vi "5668 Close Scan with External LO.vi"(8 "error in (no error)":errorcluster, 11 "Instrument Handles in":T1={"Resource Name RFSA"="RFSA", "Resource Name RFSG LO Generation"="RFSG"}) -> (0 "error out":errorcluster)   [LabVIEW 2017]
uses:
  Instrument Handles.ctl
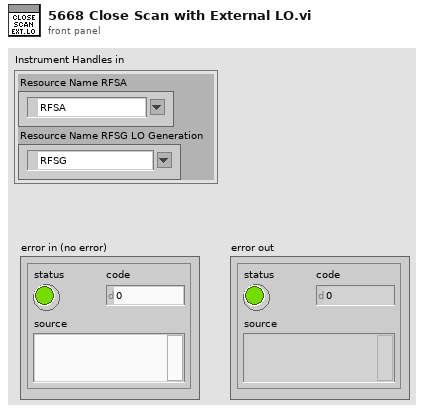
[diagram p1: front panel]
types:
  T1 = typedef "Instrument Handles.ctl" = cluster{"Resource Name RFSA":refnum<k15>, "Resource Name RFSG LO Generation":refnum<k15>}
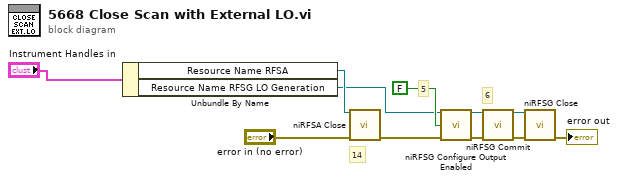
[diagram p0: block diagram]
diagram:
  # "6"
  # "5"
  # "14"
  n1 = Unbundle By Name("Instrument Handles in") -> ("Resource Name RFSA"=w4:refnum<k15>, "Resource Name RFSG LO Generation"=w3:refnum<k15>)
  n2 = call <instrlib>:"niRFSA Close.vi"("instrument handle"=w4, "error in"="error in (no error)") -> ("error out"=w2:errorcluster)  [unwired: 13 in]
  n3 = call <instrlib>:"niRFSG Configure Output Enabled.vi"("instrument handle"=w3, "output enabled"=FALSE ("output enable"), "error in"=w2) -> ("instrument handle out"=w7:refnum<k15>, "error out"=w8:errorcluster)  [unwired: 11 out]
  n4 = call <instrlib>:"niRFSG Commit.vi"("instrument handle"=w7, "error in"=w8) -> ("instrument handle out"=w10:refnum<k15>, "error out"=w9:errorcluster)  [unwired: 12 out]
  n5 = call <instrlib>:"niRFSG Close.vi"("instrument handle"=w10, "error in"=w9) -> ("error out"=→"error out":errorcluster)  [unwired: 13 out]
